vi "Save Button Info.vi"(8 "error in":errorcluster, 10 "control info":T1[](array[typedef]) {"tab level" items=["N/A", "FAB--icon--rounded", "outline--icon--rectangular", "outline--icon--rounded", "outline--text--rectangular", "outline--text--rounded", "nooutline--icon--rectangular", "nooutline--icon--rectangular--40x40", "nooutline--icon--rounded", "nooutline--text--rectangular", "nooutline--text--rounded", "tonal--icon--rectangular", "tonal--icon--rounded", "tonal--text--rectangular", "tonal--text--rounded", "filled--icon--rectangular", "filled--icon--rounded", "filled--text--rectangular", "filled--text--rounded"]; "Boolean Type" items=["N/A", "FAB--icon--rounded", "outline--icon--rectangular", "outline--icon--rounded", "outline--text--rectangular", "outline--text--rounded", "nooutline--icon--rectangular", "nooutline--icon--rectangular--40x40", "nooutline--icon--rounded", "nooutline--text--rectangular", "nooutline--text--rounded", "tonal--icon--rectangular", "tonal--icon--rounded", "tonal--text--rectangular", "tonal--text--rounded", "filled--icon--rectangular", "filled--icon--rounded", "filled--text--rectangular", "filled--text--rounded"]; "UI Theme Level" items=["N/A", "Primary", "Secondary", "Tertiary", "Error", "Primary Fixed", "Secondary Fixed", "Tertiary Fixed", "Label Only", "No Change"]}, 11 "map in":map{string, refnum<vi>}(c390)) -> (0 "error out":errorcluster)   [LabVIEW 2021]
doc: "This VI will save all of the updated tag data for the controls in the VI reference.\n\n<b>Code Developed By:</b>\nTechnology Service Corporation\nwww.tsc.com/atcs\n\nDeveloper:\nDaniel Coons"
uses:
  Material SubVIs/Material SubVIs.lvlib
  control info--typedef.ctl
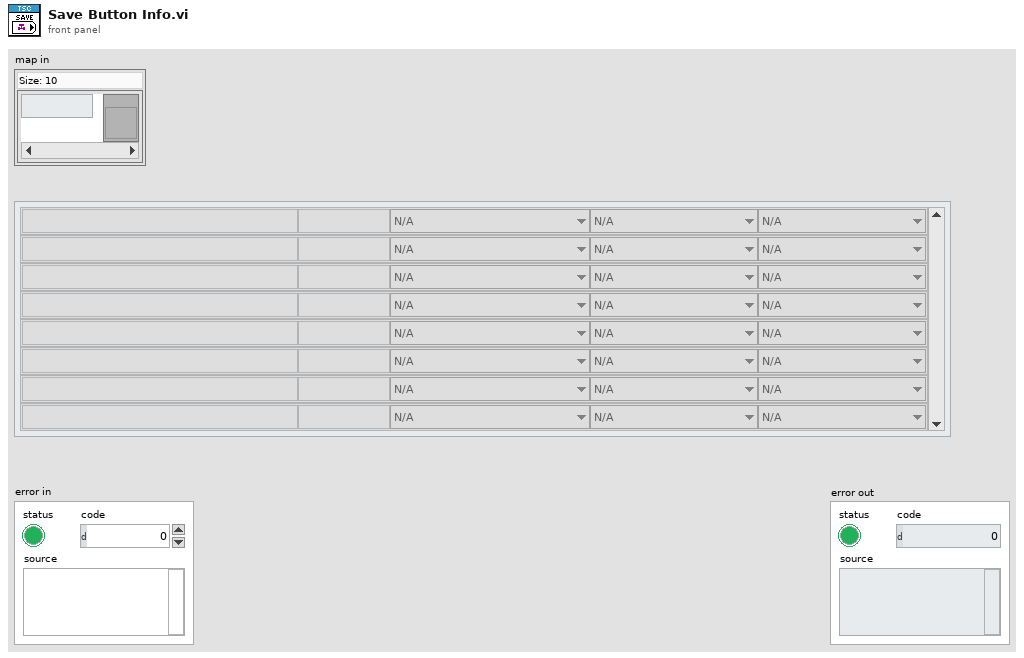
[diagram p1: front panel]
types:
  T1 = typedef "control info--typedef.ctl" = cluster{"label":string, "control type":string, "UI Theme Level":u16, "Boolean Type":u16, "tab level":u16}
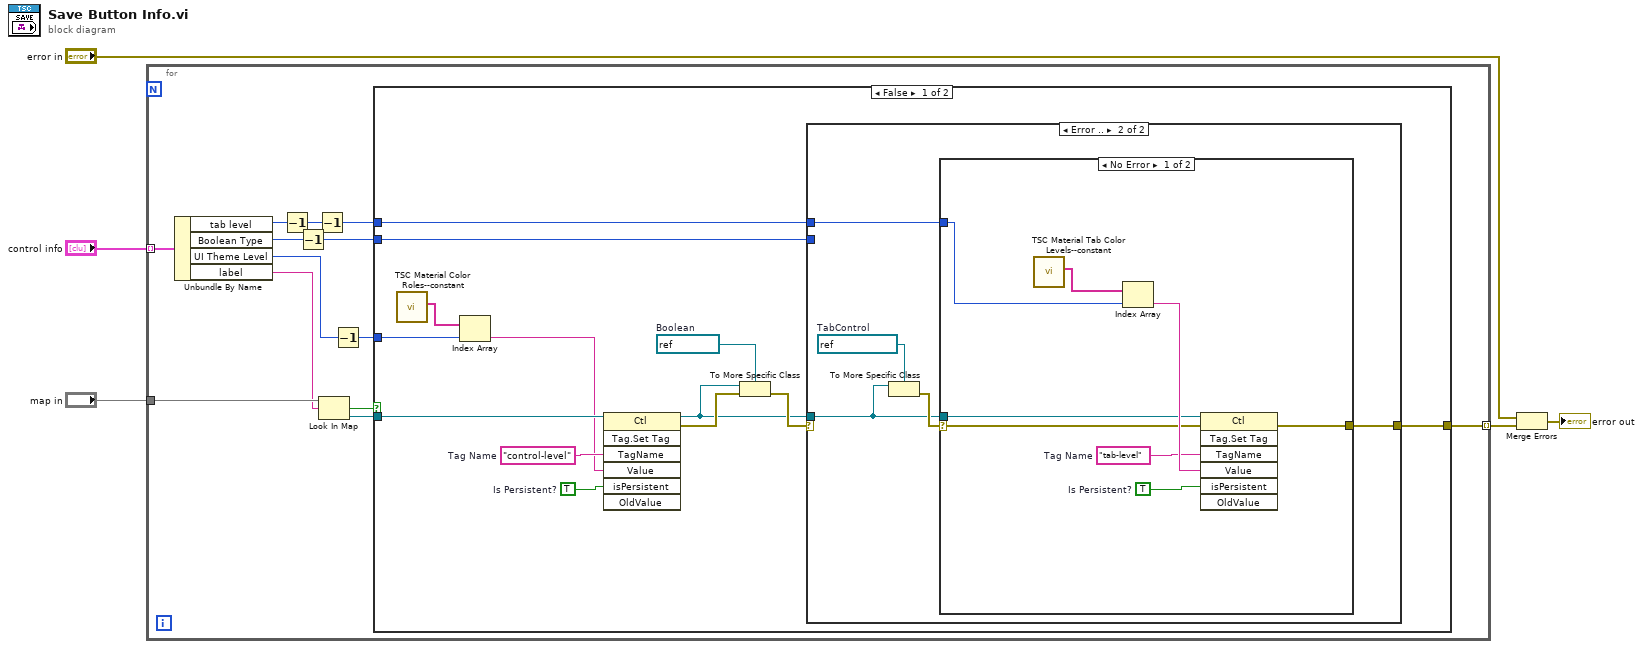
[diagram p0: block diagram]
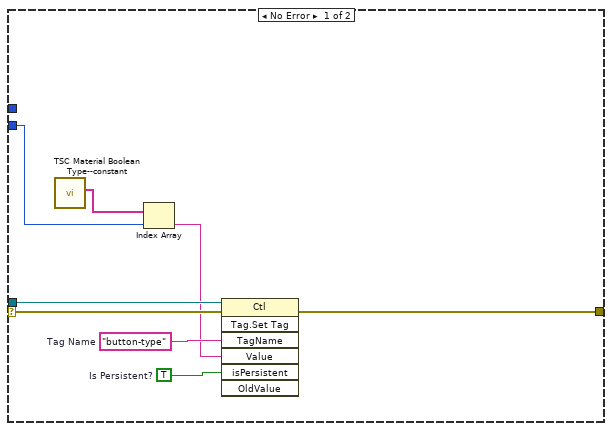
[diagram p2: hidden frame]
diagram:
  n1 = for {
    tunnel: "map in" -> [w18]
    tunnel: "control info" -> [w17] mode=indexing
    tunnel: [w11] -> w3 mode=indexing
    n2 = Unbundle By Name(w17) -> ("tab level"=w8:u16, "Boolean Type"=w12:u16, "UI Theme Level"=w13:u16, "label"=w16:string)
    n3 = Decrement(x=w8) -> (x-1=w9:u16)
    n4 = Decrement(x=w12) -> (x-1=w6:u16)
    n5 = Decrement(x=w9) -> (x-1=w7:u16)
    n6 = Look In Map(map=w18, key=w16) -> (key not found?=w15:bool, value=w14:refnum<vi>)  [unwired: 1 in]
    n7 = Decrement(x=w13) -> (x-1=w10:u16)
    n8 = case shown="False" w15 {
      tunnel: w14 -> [w27 _]
      tunnel: w10 -> [w30 _]
      tunnel: w6 -> [w20 _]
      tunnel: [w21 _] -> w11
      tunnel: w7 -> [w19 _]
      frame False {
        w24 = refnum<vi> refnum  # Boolean
        w28 = TRUE  # Is Persistent?
        w29 = "control-level"  # Tag Name
        n9 = call "TSC Material Color Roles--constant.vi"() -> ("Control Color Roles"=w31:string[])  [unwired: 11 in]
        n10 = Index Array(array=w31, index=w30) -> (element=w26:string)
        n11 = invoke class="Ctl" method="Tag.Set Tag"(reference=w27, "TagName"=w29, "Value"=w26, "isPersistent"=w28) -> (reference out=w22:refnum<vi>, error out=w25:errorcluster)  [unwired: 3 in, 5 out]
        n12 = To More Specific Class(target class=w24, reference=w22, error in=w25) -> (error out=w23:errorcluster)  [unwired: 1 out]
        n13 = case shown="Error .." w23 {
          selector: w23 -> [w38 _]
          tunnel: w22 -> [w39 w42]
          tunnel: [w37 w40] -> w21
          tunnel: w20 -> [w33 _]
          tunnel: w19 -> [_ w41]
          frame No Error {
            w35 = TRUE  # Is Persistent?
            w36 = "button-type"  # Tag Name
            n14 = call "TSC Material Boolean Type--constant.vi"() -> ("boolean types"=w34:string[])  [unwired: 11 in]
            n15 = Index Array(array=w34, index=w33) -> (element=w32:string)
            n16 = invoke class="Ctl" method="Tag.Set Tag"(reference=w39, error in=w38, "TagName"=w36, "Value"=w32, "isPersistent"=w35) -> (error out=w37:errorcluster)  [unwired: 2 in, 6 out]
          }
          frame Error {
            w44 = refnum<vi> refnum  # TabControl
            n17 = To More Specific Class(target class=w44, reference=w42) -> (error out=w43:errorcluster)  [unwired: 1 in, 1 out]
            n18 = case shown="No Error" w43 {
              selector: w43 -> [w48 _]
              tunnel: w42 -> [w47 _]
              tunnel: w41 -> [w46 _]
              tunnel: [w45 _] -> w40
              frame No Error {
                w49 = TRUE  # Is Persistent?
                w50 = "tab-level"  # Tag Name
                n19 = call "TSC Material Tab Color Levels--constant.vi"() -> ("tab color levels"=w52:string[])  [unwired: 11 in]
                n20 = Index Array(array=w52, index=w46) -> (element=w51:string)
                n21 = invoke class="Ctl" method="Tag.Set Tag"(reference=w47, error in=w48, "TagName"=w50, "Value"=w51, "isPersistent"=w49) -> (error out=w45:errorcluster)  [unwired: 2 in, 6 out]
              }
              frame Error {
              }
            }
          }
        }
      }
      frame True {
      }
    }
  }
  n22 = Merge Errors("error in", w3) -> (→"error out":errorcluster)
